vi "Search for TDMS.vi"(11 "Report Path":path) -> (1 "SystemLog":path, 2 "Found?":bool, 3 "Data File Path":path)   [LabVIEW 2018, in "File IO.lvlib"]
uses:
  File IO.lvlib
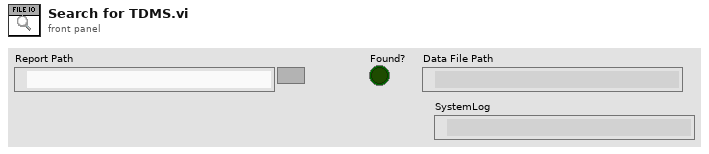
[diagram p1: front panel]
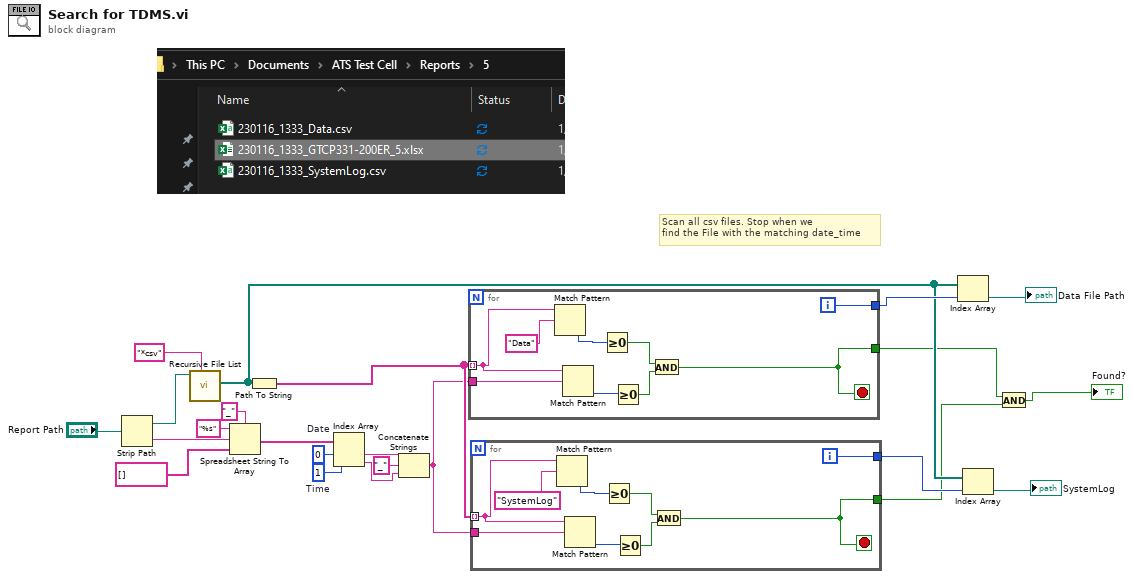
[diagram p0: block diagram]
diagram:
  w20 = 1  # Time
  w19 = 0  # Date
  # "Scan all csv files. Stop when we\nfind the File with the matching date_time"
  n1 = Strip Path(path="Report Path") -> (stripped path=w12:path, name=w15:string)
  n2 = call <vilib>:"Recursive File List.vi"("pattern"="*csv", "Folder Path"=w12) -> ("All Files in Dir"=w5:path[])  [unwired: 5 in, 4 out]
  n3 = Spreadsheet String To Array(delimiter (Tab)="_", format string="%s", spreadsheet string=w15, array type (2D Dbl)=string[] []) -> (array=w18:string[])
  n4 = Path To String(path=w5) -> (string=w8:string[])
  n5 = Index Array(array=w18, index #1=w19, index #2=w20) -> (element #1=w21:string, element #2=w23:string)
  n6 = Concatenate Strings(w21, "_" ("string"), w23) -> (w7:string)
  n7 = for {
    tunnel: w7 -> [w32]
    tunnel: w8 -> [w27] mode=indexing
    tunnel: [w30] -> w10
    tunnel: [w24] -> w3
    i -> [w30]
    stop <- w24 stop-if-true
    n8 = Match Pattern(string=w27, regular expression="Data") -> (offset past match=w28:i32)  [unwired: 1 in, 3 out]
    n9 = Match Pattern(string=w27, regular expression=w32) -> (offset past match=w31:i32)  [unwired: 1 in, 3 out]
    n10 = Greater Or Equal To 0?(x=w28) -> (x >= 0?=w26:bool)
    n11 = Greater Or Equal To 0?(x=w31) -> (x >= 0?=w25:bool)
    n12 = And(x=w26, y=w25) -> (x .and. y?=w24:bool)
  }
  n13 = for {
    tunnel: w7 -> [w41]
    tunnel: w8 -> [w36] mode=indexing
    tunnel: [w39] -> w4
    tunnel: [w33] -> w2
    i -> [w39]
    stop <- w33 stop-if-true
    n14 = Match Pattern(string=w36, regular expression="SystemLog") -> (offset past match=w37:i32)  [unwired: 1 in, 3 out]
    n15 = Match Pattern(string=w36, regular expression=w41) -> (offset past match=w40:i32)  [unwired: 1 in, 3 out]
    n16 = Greater Or Equal To 0?(x=w37) -> (x >= 0?=w35:bool)
    n17 = Greater Or Equal To 0?(x=w40) -> (x >= 0?=w34:bool)
    n18 = And(x=w35, y=w34) -> (x .and. y?=w33:bool)
  }
  n19 = Index Array(array=w5, index=w10) -> (element=→"Data File Path":path)
  n20 = Index Array(array=w5, index=w4) -> (element=→"SystemLog":path)
  n21 = And(x=w3, y=w2) -> (x .and. y?=→"Found?":bool)
